vi "currentPosition.vi"(0 "步进电机输入":refnum<visa-resource-name>) -> (1 "步进电机输出":refnum<visa-resource-name>, 2 "数值":dbl)   [LabVIEW 2018]
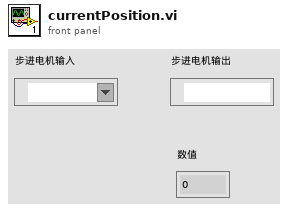
[diagram p1: front panel]
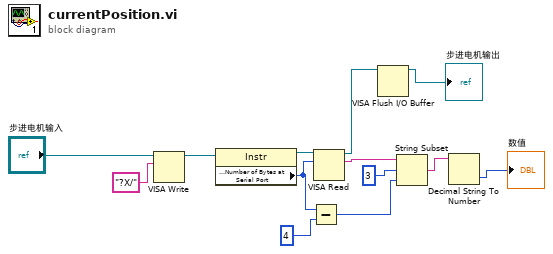
[diagram p0: block diagram]
diagram:
  n1 = VISA Write(VISA resource name="步进电机输入", write buffer="?X/") -> (VISA resource name out=w12:refnum<visa-resource-name>)  [unwired: 1 in, 2 out]
  n2 = property class="Instr"(reference=w12) -> (reference out=w11:refnum<visa-resource-name>, "Serial Settings:Number of Bytes at Serial Port"=w7:u32)  [unwired: 1 in, 1 out]
  n3 = Subtract(x=w7, y=4) -> (x-y=w6:u32)
  n4 = VISA Read(VISA resource name=w11, byte count=w7) -> (VISA resource name out=w1:refnum<visa-resource-name>, read buffer=w10:string)  [unwired: 1 in, 2 out]
  n5 = VISA Flush I/O Buffer(VISA resource name=w1) -> (VISA resource name out=→"步进电机输出":refnum<visa-resource-name>)  [unwired: 2 in, 1 out]
  n6 = String Subset(string=w10, offset (0)=3, length (rest)=w6) -> (substring=w4:string)
  n7 = Decimal String To Number(string=w4) -> (number=→"数值":i32)  [unwired: 2 in, 1 out]
